vi "create_unpack.vi"(3 "error in":errorcluster, 4 "copy? (T)":bool=TRUE, 5 "data":string) -> (0 "error out":errorcluster, 2 "u":u64)   [LabVIEW 2019, in "msgunpack.lvlib"]
doc: "Creates a msgpack unpacking object which unpacks the supplied string.\n\nNote that the string is not copied, so the string must not be deallocated until after the msgpack object has been free'd."
uses:
  msgunpack.lvlib
  msgpackalt.dll
panel:
  # "msgpack"
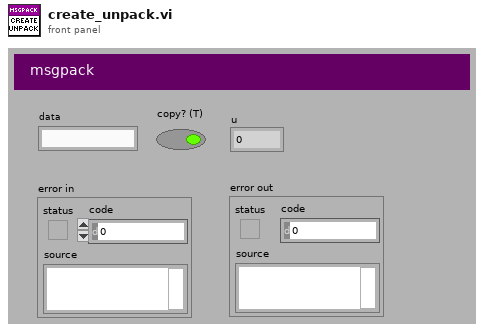
[diagram p1: front panel]
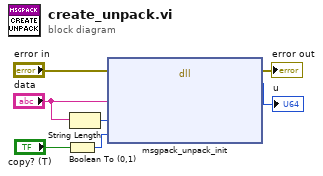
[diagram p0: block diagram]
diagram:
  n1 = Boolean To (0,1)(Boolean="copy? (T)") -> (0, 1=w1:i16)
  n2 = String Length(string="data") -> (length=w4:i32)
  n3 = dll-call lib="C:/Users/Patrick/Documents/GitHub/Instrument-Framework/lvsrc/SMOs/JSON-RPC-2019/lv-venv/lv.lib/vi.lib/addons/msgpack/msgpackalt.dll" fn="msgpack_unpack_init"(error in="error in", "data"="data", "len"=w4, "flags"=w1) -> (error out=→"error out":errorcluster, "return type"=→"u":u64)  [unwired: 5 in, 1 out]
